vi "Create Header Content Class.vi"(8 "error in (no error)":errorcluster, 11 "Simulated_Header in":refnum<class "Simulated_Header.lvclass">) -> (0 "error out":errorcluster, 3 "Simulated_Header out":refnum<class "Simulated_Header.lvclass">)   [LabVIEW 2018, in "Simulated_Header.lvclass"]
uses:
  Simulated_Header.lvclass
  Header Contents/Header Contents.lvclass
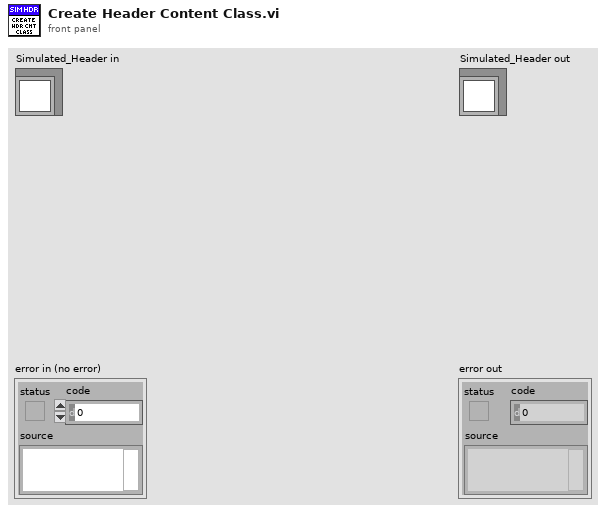
[diagram p1: front panel]
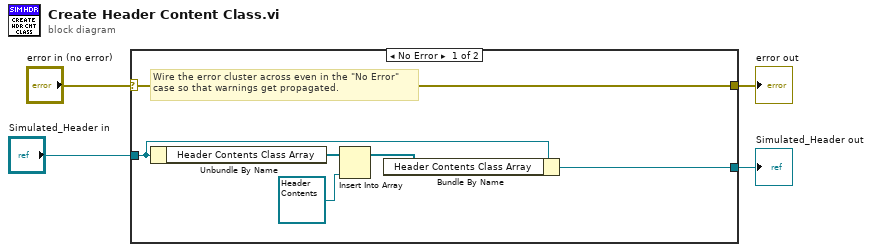
[diagram p0: block diagram]
diagram:
  n1 = case shown="No Error" "error in (no error)" {
    selector: "error in (no error)" -> [w10 w12]
    tunnel: [w10 w12] -> w3
    tunnel: [w9 w11] -> w1
    tunnel: "Simulated_Header in" -> [w8 w11]
    frame No Error {
      # "Wire the error cluster across even in the \"No Error\"\ncase so that warnings get propagated."
      n2 = Unbundle By Name(w8) -> ("Header Contents Class Array"=w7:refnum<class "Header Contents.lvclass">[])
      n3 = Insert Into Array(array=w7, new element=refnum<class "Header Contents.lvclass"> refnum ("Header Contents.lvclass")) -> (w6:refnum<class "Header Contents.lvclass">[])  [unwired: 1 in]
      n4 = Bundle By Name(cluster=w8, "Header Contents Class Array"=w6) -> (w9:refnum<class "Simulated_Header.lvclass">)
    }
    frame Error {
    }
  }
  "error out" <- w3
  "Simulated_Header out" <- w1
